vi "FFT_based_oldcode.vi"() -> ()   [LabVIEW 2020]
uses:
  <vilib>/Utility/file.llb/Read Delimited Spreadsheet (DBL).vi
panel:
  out "Computational time (ticks)":u32
  out "truth vs prediction":dbl[][](graph)
  out "Spectrum plot":cluster{i32, dbl, "spectrum out":dbl[]}(graph)
  out "Frequency Interval: delta(f)":dbl
  out "xf (frequency)":dbl[](array[numeric])
  out "size(s) 3":i32
  out "df (Hz) 3":dbl
  out "ploted signal from each selected frequency":dbl[][](graph)
  out "Input vs prediction":dbl[][](graph)
  out "truth vs prediction vs error":dbl[][](graph)
  out "Input vs prediction (zoomed)":dbl[][](graph)
  out "Time vs Acceleration \n Input learning length)":cluster{dbl[], dbl[]}[](graph)
  out "array w/ subset deleted":dbl[][](array[numeric])
  out "time":dbl[](array[numeric])
  out "Acceleration":dbl[](array[numeric])
  out "Time vs Acceleration graph(whole data)":cluster{"all rows":dbl[], "all rows":dbl[]}(graph)
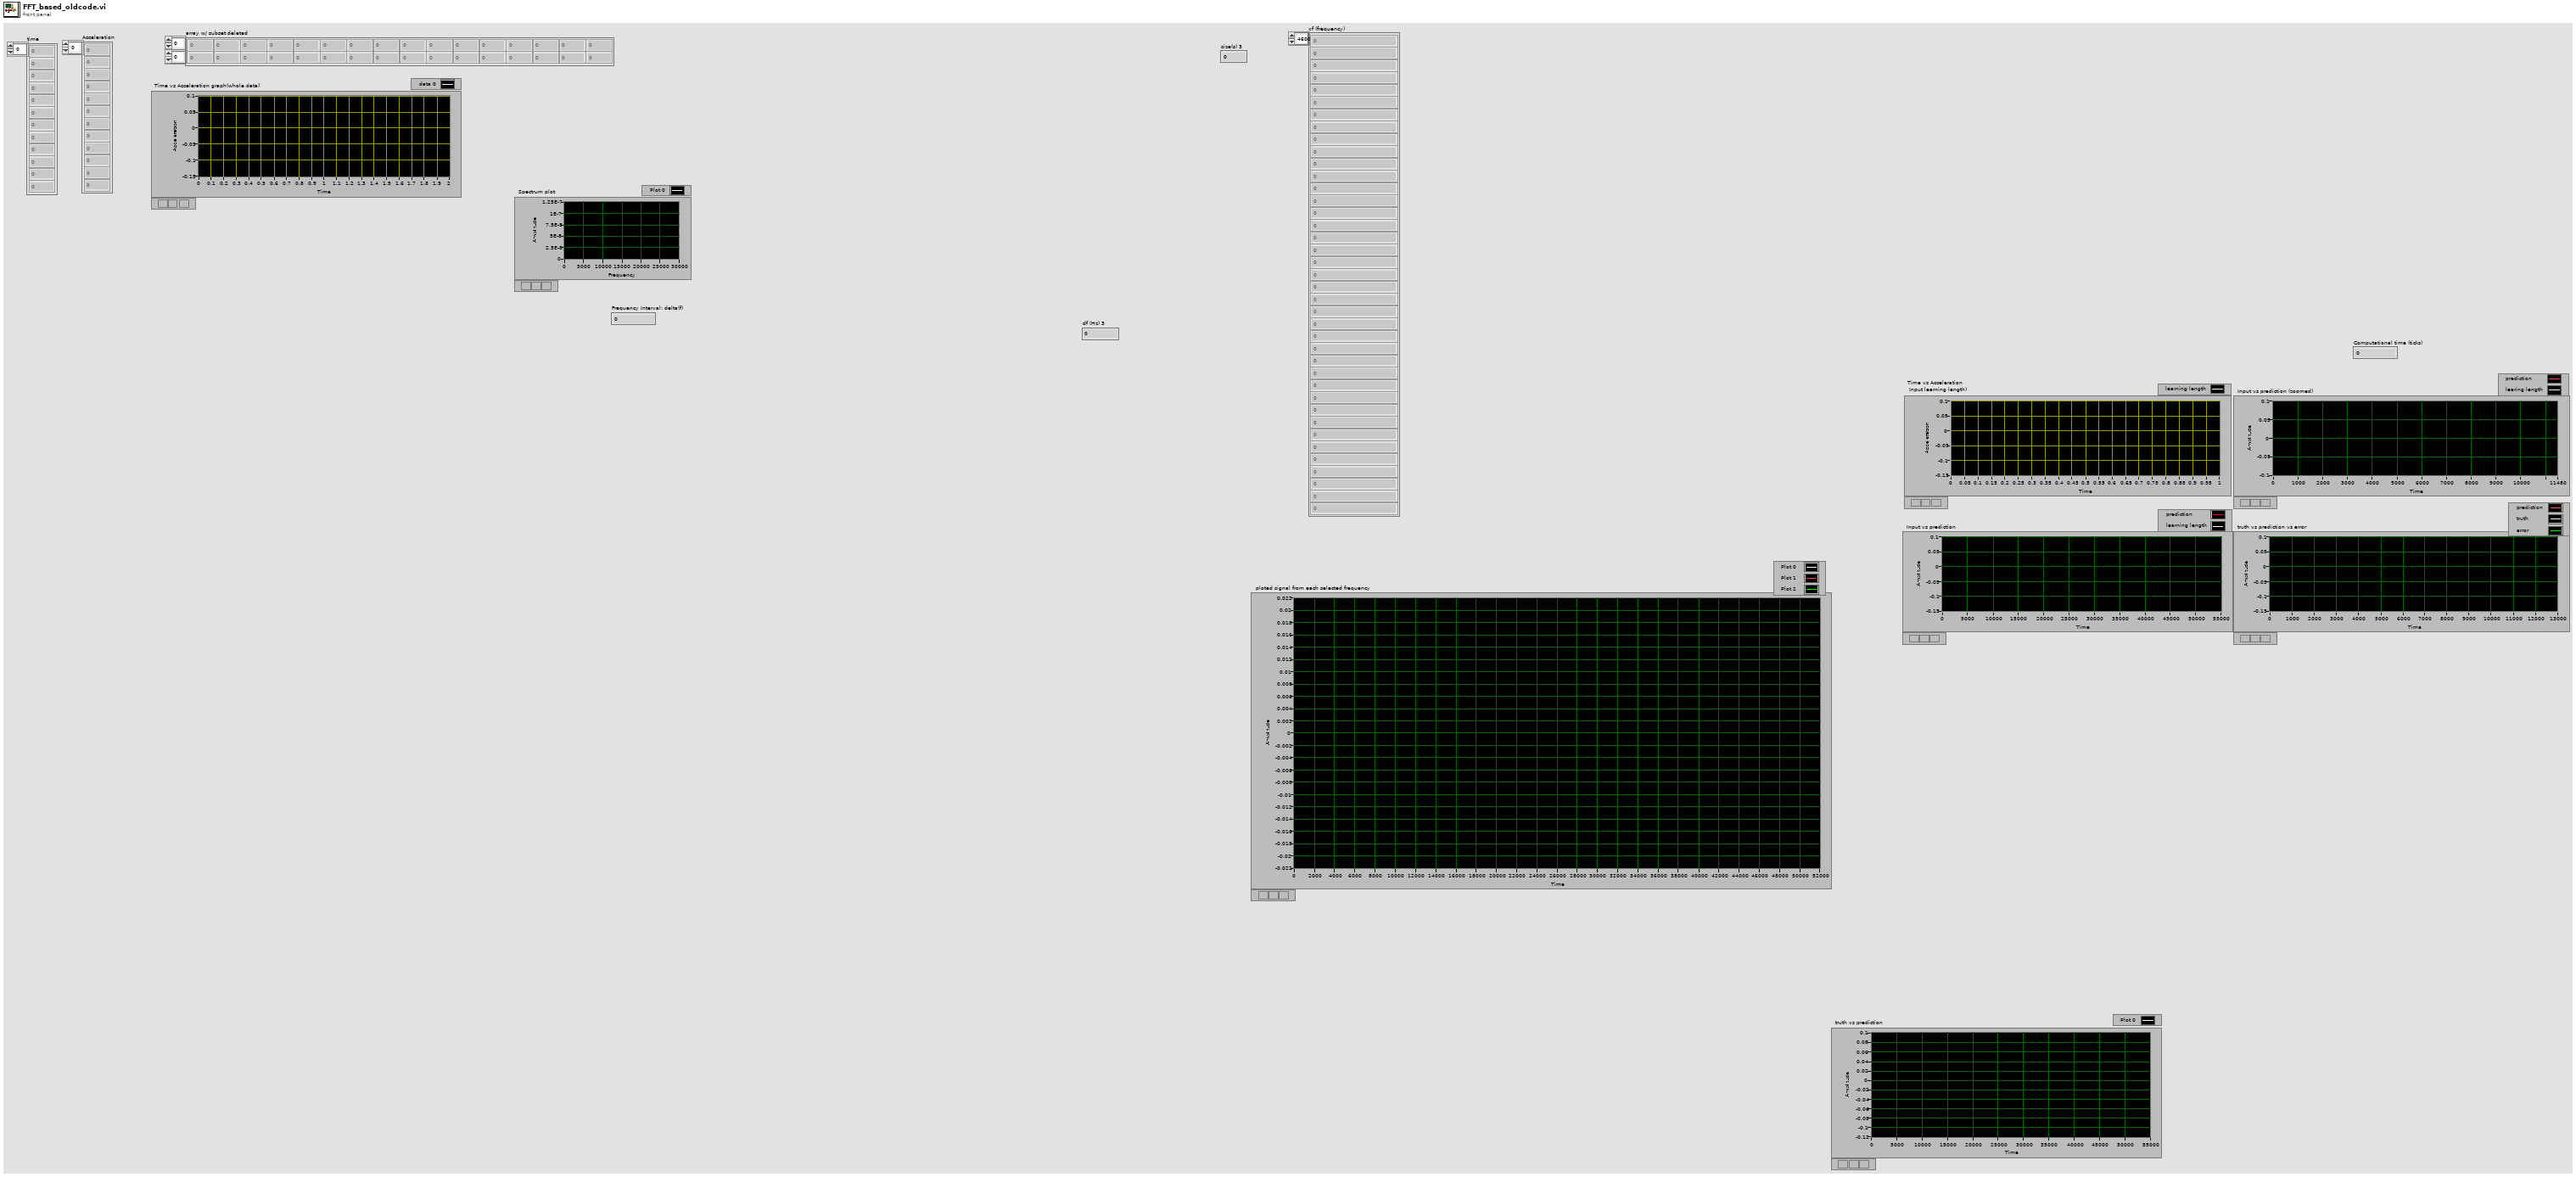
[diagram p1: front panel]
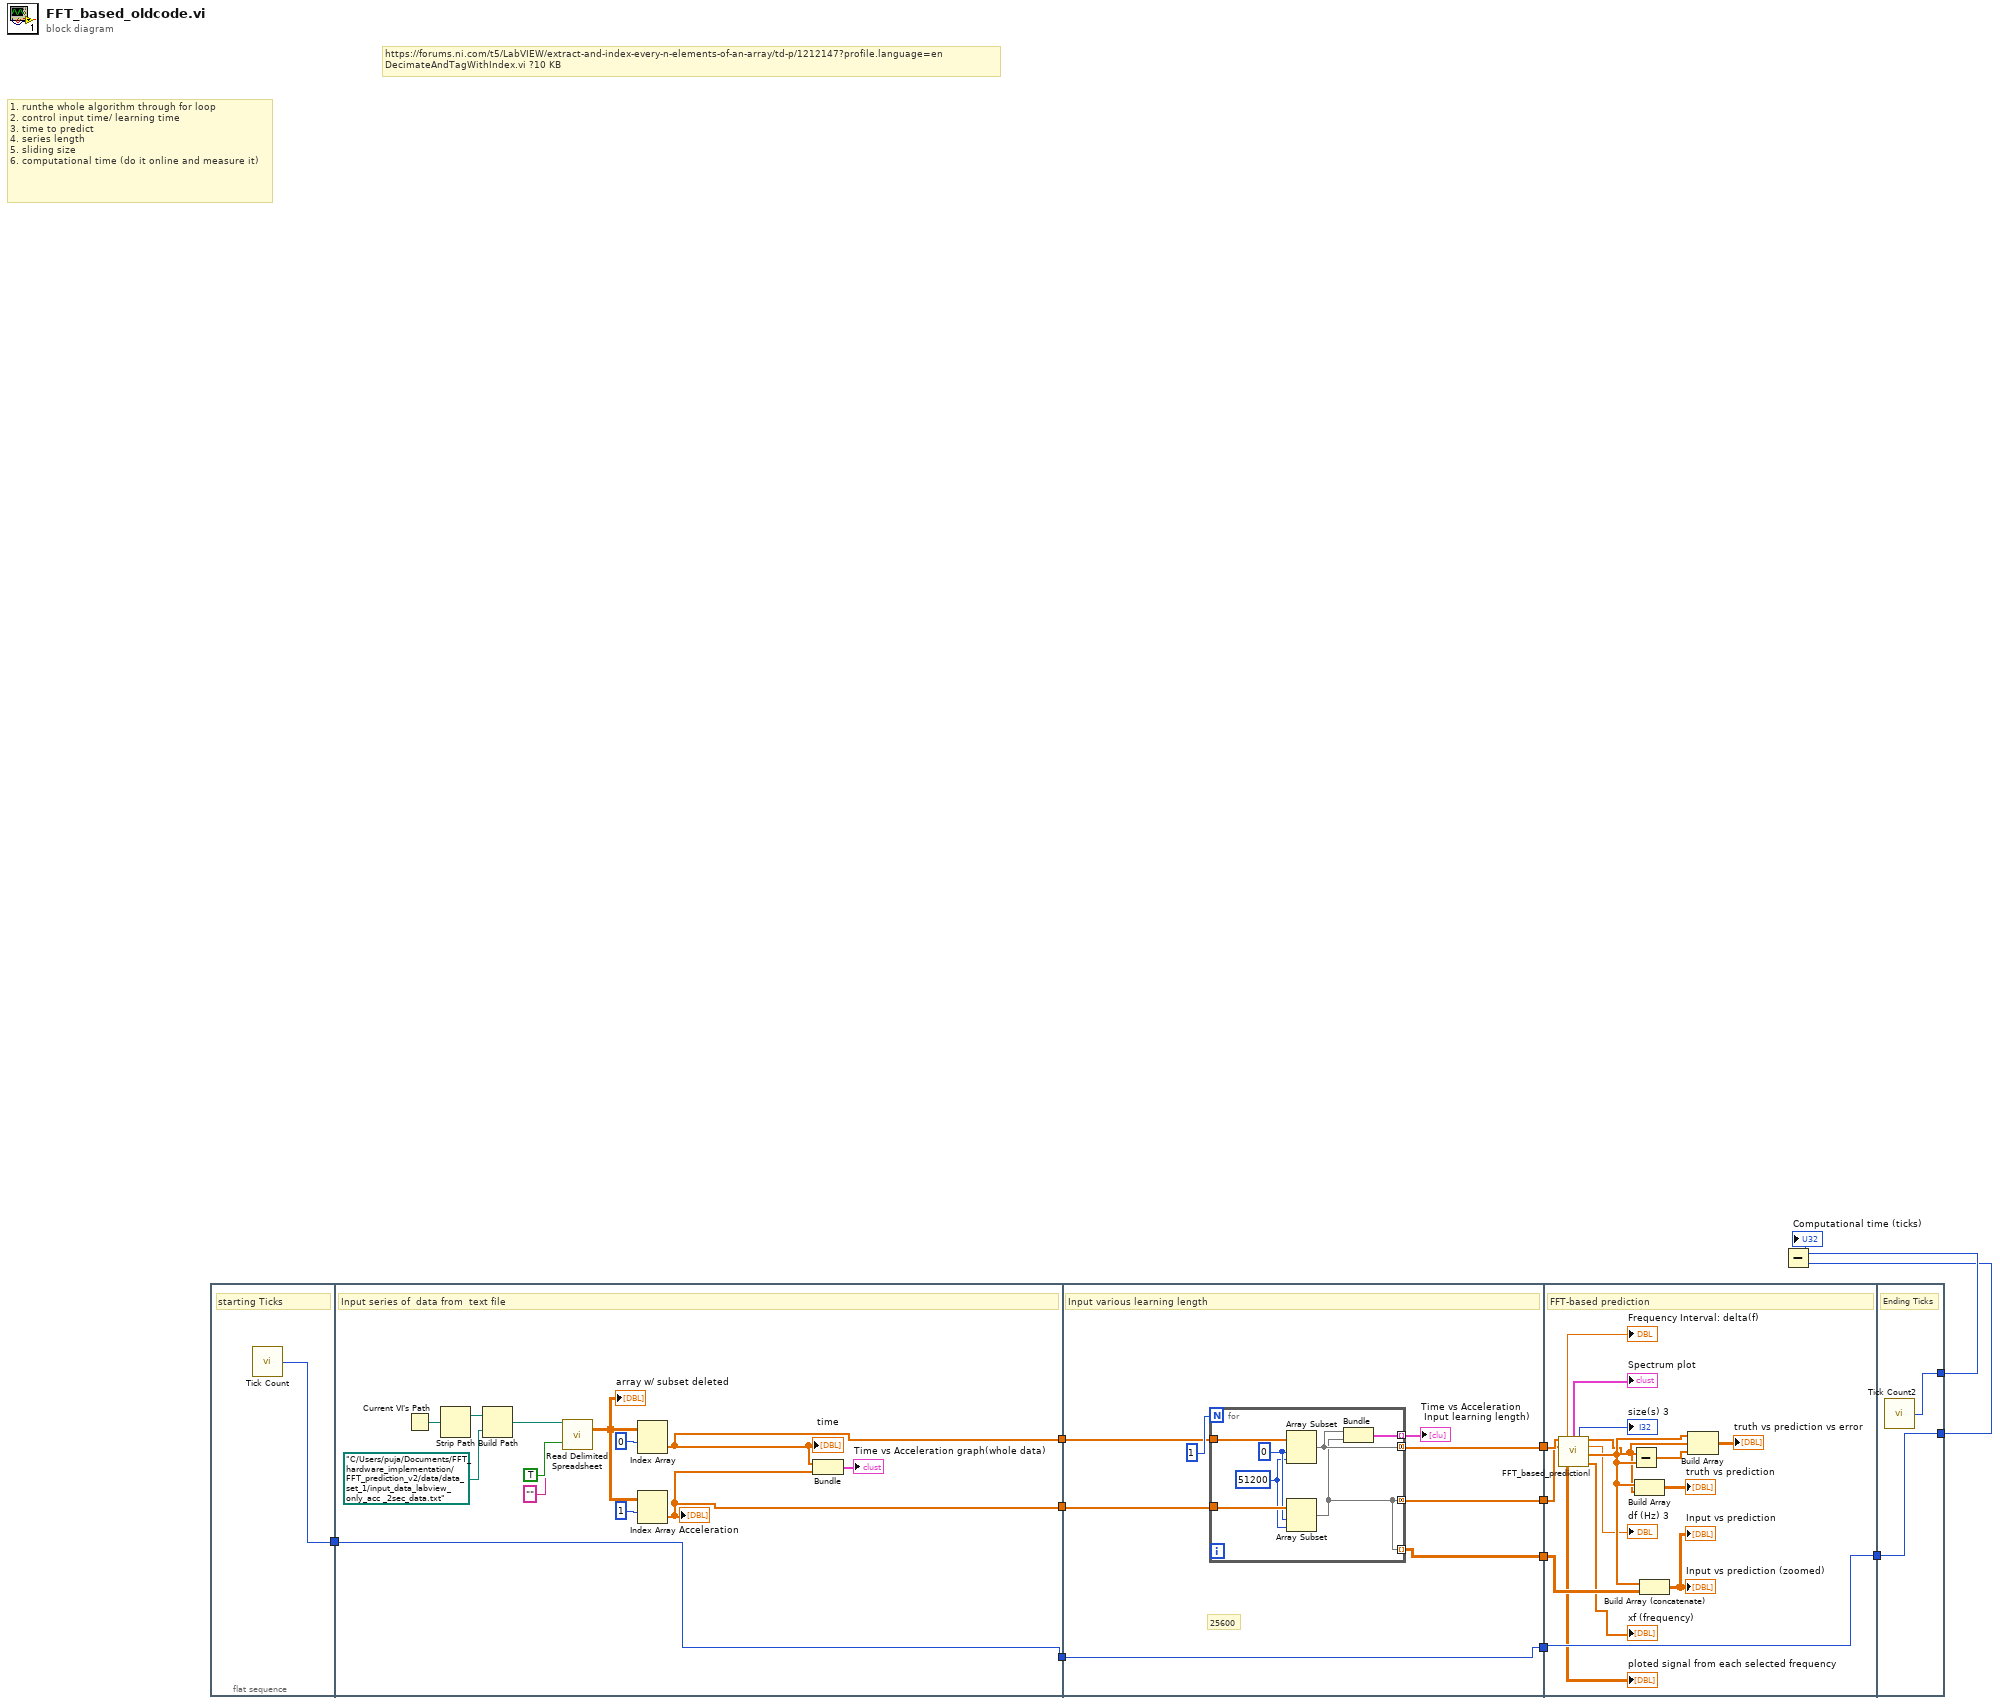
[diagram p0: block diagram]
diagram:
  # "1. runthe whole algorithm through for loop \n2. control input time/ learning time\n3. time to predict\n4. series length\n5. sliding size\n6. computational time (do it online and measure it)"
  # "https://forums.ni.com/t5/LabVIEW/extract-and-index-every-n-elements-of-an-array/td-p/1212147?profile.language=en\nDecimateAndTagWithIndex.vi ?10 KB"
  n1 = flat-sequence {
    tunnel: [w13] -> w12
    tunnel: [w17] -> w11
    tunnel: [w16] -> w10
    tunnel: [w14] -> w9
    tunnel: w12 -> [w14]
    tunnel: w11 -> [w33]
    tunnel: w10 -> [w32]
    tunnel: [w30] -> w8
    tunnel: [w29] -> w7
    tunnel: [w28] -> w6
    tunnel: w9 -> [w27]
    tunnel: [w27] -> w5
    tunnel: w8 -> [w50]
    tunnel: w7 -> [w49]
    tunnel: w6 -> [w53]
    tunnel: w5 -> [w52]
    tunnel: [w52] -> w4
    tunnel: [w59] -> w3
    tunnel: w4 -> [w58]
    tunnel: [w58] -> w2
    frame #0 {
      # "starting Ticks"
      n2 = call "Tick Count"() -> ("Tick Count(uSec)"=w13:u32)
    }
    frame #1 {
      # "Input series of  data from  text file"
      n3 = Current VI's Path() -> (path=w24:path)
      n4 = Strip Path(path=w24) -> (stripped path=w25:path)  [unwired: 1 out]
      n5 = Build Path(base path=w25, name or relative path=path "C:/Users/puja/Documents/FFT_hardware_implementation/FFT_prediction_v2/data/data_set_1/input_data_labview_only_acc _2sec_data.txt") -> (appended path=w26:path)
      n6 = call-poly <vilib>:"Read Delimited Spreadsheet.vi"("file path (dialog if empty)"=w26, "transpose? (F)"=TRUE, "delimiter (\\t)"="" ("delimiter (\\t)")) -> ("all rows"=w23:dbl[][])  [unwired: 7 in, 5 out]
      "array w/ subset deleted" <- w23
      n7 = Index Array(array=w23, index (row)=0) -> (element=w17:dbl[])  [unwired: 1 in]
      "time" <- w17
      n8 = Index Array(array=w23, index (row)=1) -> (element=w16:dbl[])  [unwired: 1 in]
      "Acceleration" <- w16
      n9 = Bundle("all rows"=w17, "all rows"=w16) -> (→"Time vs Acceleration graph(whole data)":cluster{"all rows":dbl[], "all rows":dbl[]})  [unwired: 1 in]
    }
    frame #2 {
      # "25600"
      # "Input various learning length"
      n10 = for {
        N: 1 -> [_]
        tunnel: w33 -> [w41]
        tunnel: [w38] -> w30 mode=concatenating
        tunnel: w32 -> [w40]
        tunnel: [w36] -> w29 mode=concatenating
        tunnel: [w37] -> w31 mode=indexing
        tunnel: [w36] -> w28 mode=indexing
        w39 = 0
        w35 = 51200 ("length")
        n11 = Array Subset(array=w41, index=w39, length=w35) -> (w38:dbl[])
        n12 = Array Subset(array=w40, index=w39, length=w35) -> (w36:dbl[])
        n13 = Bundle(w38, w36) -> (w37:cluster{dbl[], dbl[]})  [unwired: 1 in]
      }
      "Time vs Acceleration \n Input learning length)" <- w31
    }
    frame #3 {
      # "FFT-based prediction"
      n14 = call "FFT_based_predictionl.vi"("time"=w50, "acceleration"=w49) -> ("Frequency Interval: delta(f)"=→"Frequency Interval: delta(f)":dbl, "Spectrum plot"=→"Spectrum plot":cluster{i32, dbl, "spectrum out":dbl[]}, "size(s)"=→"size(s) 3":i32, "all rows"=w42:dbl[], "df (Hz)"=→"df (Hz) 3":dbl, "xf (frequency)"=w44:dbl[], "ploted signal from each selected frequency"=→"ploted signal from each selected frequency":dbl[][], "magnitude 2"=→"xf (frequency)":dbl[])  [unwired: 4 in, 2 out]
      n15 = Subtract(x=w42, y=w44) -> (x-y=w56:dbl[])
      n16 = Build Array(w44, w42) -> (→"truth vs prediction":dbl[][])
      n17 = Build Array (concatenate)(w44, w53) -> (→"Input vs prediction" →"Input vs prediction (zoomed)":dbl[][])
      n18 = Build Array(w44, w42, w56) -> (→"truth vs prediction vs error":dbl[][])
    }
    frame #4 {
      # "Ending Ticks"
      n19 = call "Tick Count2"() -> ("Tick Count(uSec)"=w59:u32)
    }
  }
  n20 = Subtract(x=w3, y=w2) -> (x-y=→"Computational time (ticks)":u32)
